vi "打开数据记录文件.vi"(8 "错误输入":errorcluster, 11 "路径in":path) -> (0 "error out":errorcluster, 3 "引用句柄输出":refnum<file>)   [LabVIEW 2020]
panel:
  out "大小（字节）":i64
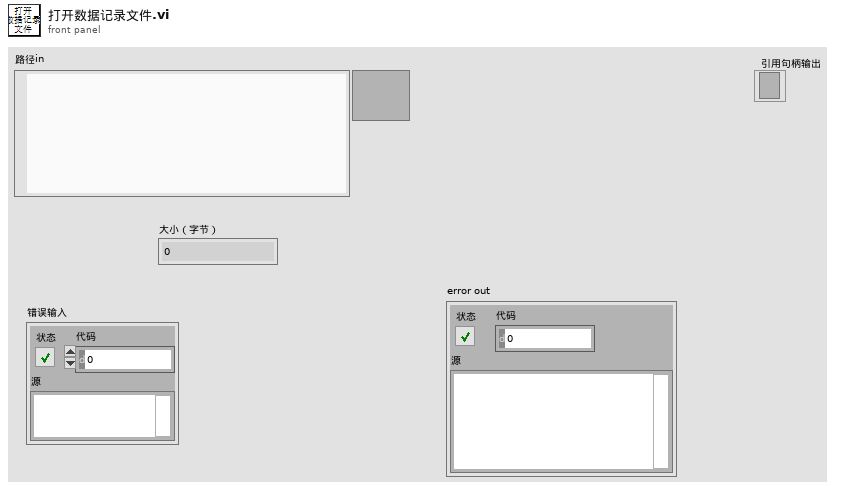
[diagram p1: front panel]
types:
  T1 = enum16{"open", "replace", "create", "open or create", "replace or create", "replace or create with confirmation"}
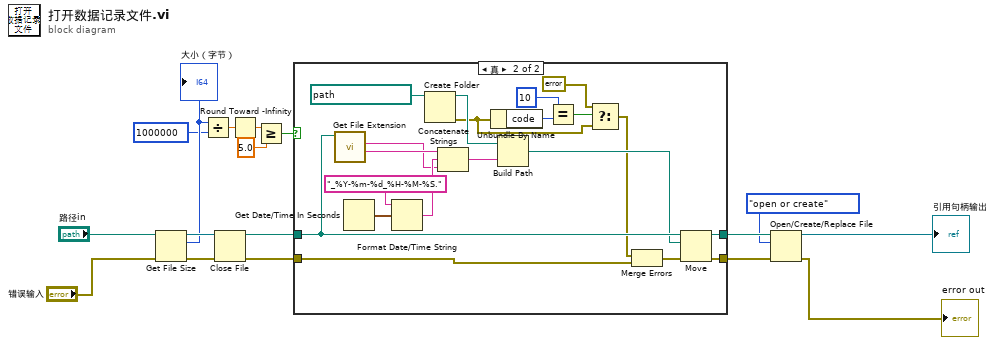
[diagram p0: block diagram]
diagram:
  n1 = Get File Size(file="路径in", error in="错误输入") -> (refnum out=w17:refnum<file>, size (in bytes)=w15:i64, 0:w16:errorcluster)
  "大小（字节）" <- w15
  n2 = Divide(x=w15, y=i64 1000000) -> (x/y=w13:dbl)
  n3 = Close File(refnum=w17, error in=w16) -> (path=w9:path, error out=w8:errorcluster)
  n4 = Round Toward -Infinity(1:w13) -> (0:w12:dbl)
  n5 = Greater Or Equal?(x=w12, y=5.0) -> (x >= y?=w10:bool)
  n6 = case shown="真" w10 {
    tunnel: w9 -> [w19 w39]
    tunnel: w8 -> [w18 w24]
    tunnel: [w19 w32] -> w5
    tunnel: [w18 w31] -> w3
    frame False {
    }
    frame True {
      n7 = call <vilib>:"Get File Extension.vi"("file"=w39) -> ("filename without extension"=w36:string, "lowercase file extension"=w34:string)  [unwired: 6 in, 3 out]
      n8 = Get Date/Time In Seconds() -> (seconds since 1Jan1904=w38:timestamp)
      n9 = Format Date/Time String(time format string (%c)="_%Y-%m-%d_%H-%M-%S." ("时间格式字符串(%c)"), seconds (now)=w38) -> (date/time string=w35:string)  [unwired: 1 in]
      n10 = Create Folder(path (use dialog)=path "D:/气压数据Bak" ("路径in")) -> (created path=w29:path, error out=w23:errorcluster)  [unwired: 2 in, 1 out]
      n11 = Concatenate Strings(w36, w35, w34) -> (w33:string)
      n12 = Unbundle By Name(w23) -> ("code"=w27:i32)
      n13 = Build Path(base path=w29, name or relative path=w33) -> (appended path=w28:path)
      n14 = Equal?(x=10, y=w27) -> (x = y?=w25:bool)
      n15 = Select(t=errorcluster {"status"=FALSE, "code"=0, "source"=""} ("error out"), s=w25, f=w23) -> (s? t:f=w20:errorcluster)
      n16 = Merge Errors(w20, w24) -> (w21:errorcluster)
      n17 = Move(source path=w39, error in=w21, 10:w28) -> (error out=w31:errorcluster, 3:w32:path)  [unwired: 2 in, 1 out]
    }
  }
  n18 = Open/Create/Replace File(file path (use dialog)=w5, error in=w3, operation (0:open)=T1."open or create" ("操作(0:open)")) -> (refnum out=→"引用句柄输出":refnum<file>, error out=→"error out":errorcluster)  [unwired: 3 in, 1 out]
